vi "Write Scale.vi"(8 "error in (no error)":errorcluster, 10 "Scale (V/LSB)":dbl[](array[numeric]), 11 "AcquireTraces in":refnum<class "AcquireTraces.lvclass">) -> (0 "error out":errorcluster, 3 "AcquireTraces out":refnum<class "AcquireTraces.lvclass">)   [LabVIEW 2014, in "AcquireTraces.lvclass"]
uses:
  AcquireTraces.lvclass
  AcquireTraces.lvclass/AcquireTraces.ctl
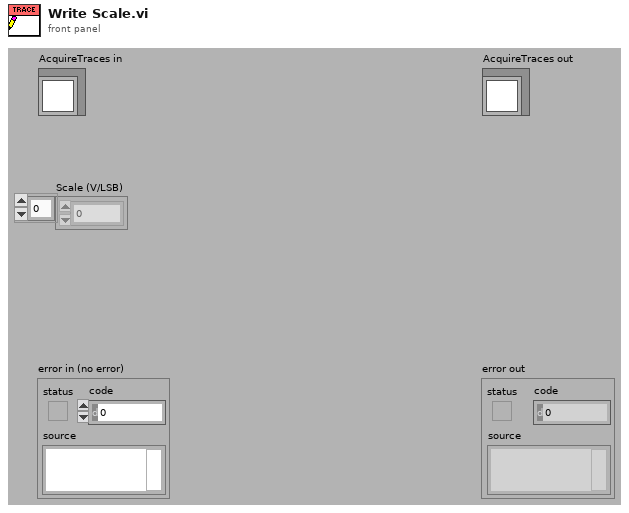
[diagram p1: front panel]
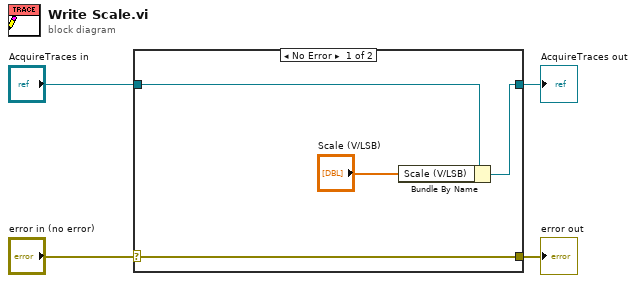
[diagram p0: block diagram]
diagram:
  n1 = case shown="No Error" "error in (no error)" {
    selector: "error in (no error)" -> [w8 w9]
    tunnel: [w8 w9] -> w3
    tunnel: [w6 w10] -> w1
    tunnel: "AcquireTraces in" -> [w7 w10]
    frame No Error {
      n2 = Bundle By Name(cluster=w7, "Scale (V/LSB)"="Scale (V/LSB)") -> (w6:refnum<class "AcquireTraces.lvclass">)
    }
    frame Error {
    }
  }
  "error out" <- w3
  "AcquireTraces out" <- w1
